vi "KE622x -- DCon Mode Set Params.vi"(0 "Resource In":refnum<visa-resource-name>, 1 "Check For SCPI Errors? (T)":bool=TRUE, 7 "Differential Cond Params In":T2={"Start Value (A)"=0.0, "Stop Value (A)"=-1e-05, "Step Size (A)"=1e-05, "Delta Value (A)"=1e-06, "Delay (s)"=1e-06, "Abort On\nCompliance?"=FALSE} {"Delay (s)" min=0.001 max=9999.999 format="%.3f"; "Delta Value (A)" min=0.0 max=0.105 format="%.3p"; "Step Size (A)" min=0.0 max=0.105 format="%.3p"; "Stop Value (A)" min=-0.105 max=0.105 format="%.3p"; "Start Value (A)" min=-0.105 max=0.105 format="%.3p"}, 11 "error in (no error)":errorcluster, 12 "Read Back Set Values? (T)":bool=TRUE) -> (4 "Resource Out (dupl)":refnum<visa-resource-name>, 8 "Differential Cond Params Out":T2={"Start Value (A)"=0.0, "Stop Value (A)"=-1e-05, "Step Size (A)"=1e-05, "Delta Value (A)"=1e-06, "Delay (s)"=1e-06, "Abort On\nCompliance?"=FALSE} {"Delay (s)" min=0.001 max=9999.999 format="%.3f"; "Delta Value (A)" min=0.0 max=0.105 format="%.3p"; "Step Size (A)" min=0.0 max=0.105 format="%.3p"; "Stop Value (A)" min=-0.105 max=0.105 format="%.3p"; "Start Value (A)" min=-0.105 max=0.105 format="%.3p"}, 13 "Num Buf Points":u32, 14 "Last Buf Point Source Value (A)":T1=-1e-05 min=-0.105 max=0.105 format="%.3p", 15 "error out":errorcluster)   [LabVIEW 2010, in "Keithley 622x.lvlib"]
doc: "Sets the parameters for 'Differntial Conductance' measurements. Note that performing this measurement implies that the 622x is being used in conjuction with a 2182/2182A nano-voltmeter."
uses:
  Keithley 622x.lvlib
  Low Level/Typedefs/KE622x -- DCon Mode Start Stop Level.ctl
  Low Level/Typedefs/KE622x -- DCon Mode Step Delta Size.ctl
  Low Level/Typedefs/KE622x -- Delta DCon Mode Delay.ctl
  Typedefs/KE622x -- DCon Mode Params.ctl
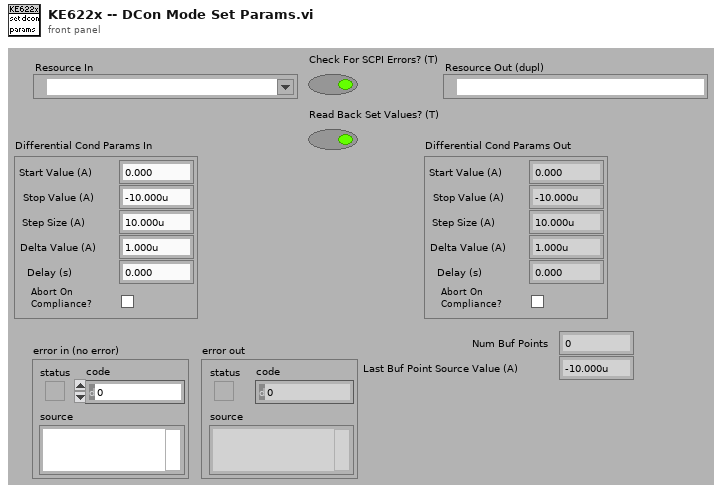
[diagram p1: front panel]
types:
  T1 = typedef "Keithley 622x.lvlib/KE622x -- DCon Mode Start Stop Level.ctl" = dbl
  T2 = typedef "Keithley 622x.lvlib/KE622x -- DCon Mode Params.ctl" = cluster{"Start Value (A)":T1, "Stop Value (A)":T1, "Step Size (A)":T3, "Delta Value (A)":T3, "Delay (s)":T4, "Abort On\nCompliance?":bool}
  T3 = typedef "Keithley 622x.lvlib/KE622x -- DCon Mode Step Delta Size.ctl" = dbl
  T4 = typedef "Keithley 622x.lvlib/KE622x -- Delta DCon Mode Delay.ctl" = dbl
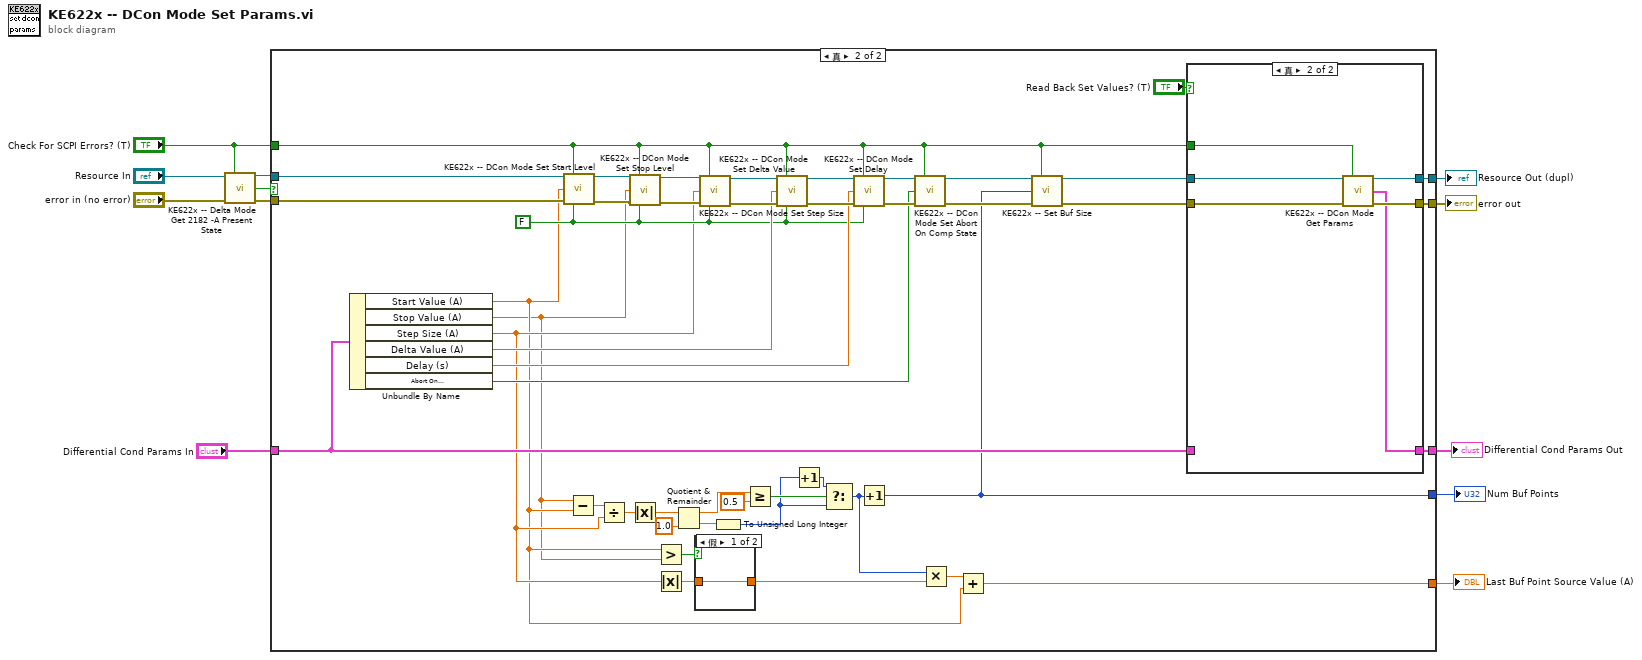
[diagram p0: block diagram]
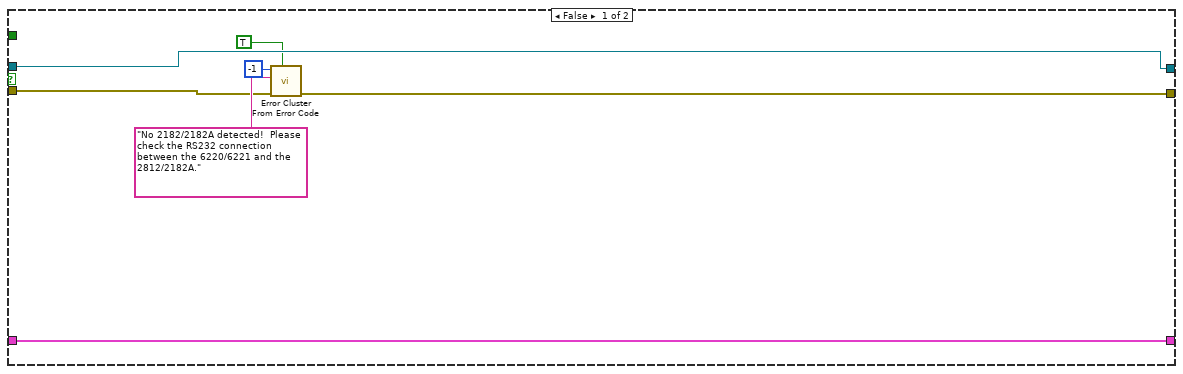
[diagram p2: hidden frame]
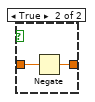
[diagram p3: hidden frame]
diagram:
  n1 = call "KE622x -- Delta Mode Get 2182 -A Present State.vi"("Resource In"="Resource In", "Check For SCPI Errors? (T)"="Check For SCPI Errors? (T)", "error in (no error)"="error in (no error)") -> ("Resource Out (dupl)"=w8:refnum<visa-resource-name>, "2182/2182A Present?"=w6:bool, "error out"=w7:errorcluster)  [unwired: 10 in]
  n2 = case shown="真" w6 {
    tunnel: w8 -> [w15 w65]
    tunnel: w7 -> [w17 w64]
    tunnel: [w15 w52] -> w12
    tunnel: [w16 w51] -> w11
    tunnel: "Differential Cond Params In" -> [w14 w50]
    tunnel: [w14 w49] -> w3
    tunnel: "Check For SCPI Errors? (T)" -> [_ w21]
    tunnel: [_ w20] -> w2
    tunnel: [_ w27] -> w1
    frame False {
      n3 = call <vilib>:"Error Cluster From Error Code.vi"("show call chain? (False)"=TRUE, "error in (no error)"=w17, "error message (\"\")"="No 2182/2182A detected!  Please check the RS232 connection between the 6220/6221 and the 2812/2182A.", "error code (0)"=-1) -> ("error out"=w16:errorcluster)  [unwired: 5 in]
    }
    frame True {
      w45 = FALSE ("Read Back Set Value? (T)")
      n4 = Unbundle By Name(w50) -> ("Start Value (A)"=w28:T1, "Stop Value (A)"=w26:T1, "Step Size (A)"=w33:T3, "Delta Value (A)"=w48:T3, "Delay (s)"=w47:T4, "Abort On\nCompliance?"=w46:bool)
      n5 = call <instrlib>:"KE622x -- DCon Mode Set Start Level.vi"("Resource In"=w65, "Check For SCPI Errors? (T)"=w21, "Start Level In (A)"=w28, "error in (no error)"=w64, "Read Back Set Value? (T)"=w45) -> ("Resource Out (dupl)"=w63:refnum<visa-resource-name>, "error out"=w62:errorcluster)  [unwired: 8 in, 1 out]
      n6 = Subtract(x=w26, y=w28) -> (x-y=w42:T1)
      n7 = Divide(x=w42, y=w33) -> (x/y=w44:T1)
      n8 = call "KE622x -- DCon Mode Set Stop Level.vi"("Resource In"=w63, "Check For SCPI Errors? (T)"=w21, "Stop Level In (A)"=w26, "error in (no error)"=w62, "Read Back Set Value? (T)"=w45) -> ("Resource Out (dupl)"=w61:refnum<visa-resource-name>, "error out"=w60:errorcluster)  [unwired: 8 in, 1 out]
      n9 = Absolute Value(x=w44) -> (abs(x)=w41:T1)
      n10 = Greater?(x=w28, y=w26) -> (0:w34:bool)
      n11 = Absolute Value(x=w33) -> (abs(x)=w32:T3)
      n12 = Quotient & Remainder(x=w41, y=T1 1.0) -> (x-y*floor(x/y)=w39:T1, floor(x/y)=w40:T1)
      n13 = case shown="假" w34 {
        tunnel: w32 -> [w66 w68]
        tunnel: [w66 w67] -> w31
        frame False {
        }
        frame True {
          n14 = Negate(x=w68) -> (-x=w67:T3)
        }
      }
      n15 = call <instrlib>:"KE622x -- DCon Mode Set Step Size.vi"("Resource In"=w61, "Check For SCPI Errors? (T)"=w21, "Step Size In (A)"=w33, "error in (no error)"=w60, "Read Back Set Value? (T)"=w45) -> ("Resource Out (dupl)"=w59:refnum<visa-resource-name>, "error out"=w58:errorcluster)  [unwired: 8 in, 1 out]
      n16 = To Unsigned Long Integer(number=w40) -> (unsigned 32bit integer=w36:u32)
      n17 = Greater Or Equal?(x=w39, y=T1 0.5) -> (x >= y?=w37:bool)
      n18 = call "KE622x -- DCon Mode Set Delta Value.vi"("Resource In"=w59, "Check For SCPI Errors? (T)"=w21, "Delta Value In (A)"=w48, "error in (no error)"=w58, "Read Back Set Value? (T)"=w45) -> ("Resource Out (dupl)"=w55:refnum<visa-resource-name>, "error out"=w54:errorcluster)  [unwired: 8 in, 1 out]
      n19 = Increment(x=w36) -> (x+1=w35:u32)
      n20 = Select(t=w35, s=w37, f=w36) -> (s? t:f=w30:u32)
      n21 = call <instrlib>:"KE622x -- DCon Mode Set Delay.vi"("Resource In"=w55, "Check For SCPI Errors? (T)"=w21, "Delay In (s)"=w47, "error in (no error)"=w54, "Read Back Set Value? (T)"=w45) -> ("Resource Out (dupl)"=w57:refnum<visa-resource-name>, "error out"=w56:errorcluster)  [unwired: 8 in, 1 out]
      n22 = Increment(x=w30) -> (x+1=w20:u32)
      n23 = call "KE622x -- DCon Mode Set Abort On Comp State.vi"("Resource In"=w57, "Check For SCPI Errors? (T)"=w21, "Abort On Compliance?"=w46, "error in (no error)"=w56) -> ("Resource Out (dupl)"=w24:refnum<visa-resource-name>, "error out"=w25:errorcluster)  [unwired: 10 in]
      n24 = Multiply(x=w30, y=w31) -> (x*y=w29:T3)
      n25 = Add(x=w29, y=w28) -> (x+y=w27:T3)
      n26 = call <instrlib>:"KE622x -- Set Buf Size.vi"("Resource In"=w24, "Check For SCPI Errors? (T)"=w21, "Buffer Size (Num Readings)"=w20, "error in (no error)"=w25) -> ("Resource Out (dupl)"=w22:refnum<visa-resource-name>, "error out"=w23:errorcluster)  [unwired: 10 in]
      n27 = case shown="真" "Read Back Set Values? (T)" {
        tunnel: w22 -> [w71 w77]
        tunnel: w23 -> [w70 w76]
        tunnel: [w71 w75] -> w52
        tunnel: [w70 w74] -> w51
        tunnel: w50 -> [w69 _]
        tunnel: [w69 w73] -> w49
        tunnel: w21 -> [_ w72]
        frame False {
        }
        frame True {
          n28 = call "KE622x -- DCon Mode Get Params.vi"("Resource In"=w77, "Check For SCPI Errors? (T)"=w72, "error in (no error)"=w76) -> ("Resource Out (dupl)"=w75:refnum<visa-resource-name>, "Differential Cond Params"=w73:T2, "error out"=w74:errorcluster)  [unwired: 10 in]
        }
      }
    }
  }
  "Resource Out (dupl)" <- w12
  "error out" <- w11
  "Differential Cond Params Out" <- w3
  "Num Buf Points" <- w2
  "Last Buf Point Source Value (A)" <- w1
